vi "FolderMon start.vi"(4 "error in (no error)":errorcluster, 7 "daemon VI ref":refnum<vi>) -> (0 "error out":errorcluster, 3 "dup daemon VI ref":refnum<vi>)   [LabVIEW 2011]
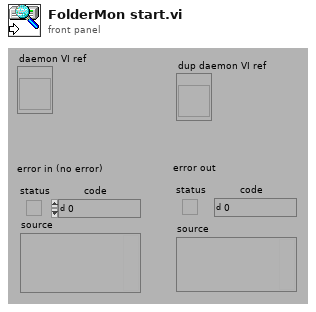
[diagram p1: front panel]
types:
  T1 = enum32{"Bad", "Idle", "Run top level", "Running"}
  T2 = typedef "Rendezvous RefNum" = refnum<k1>
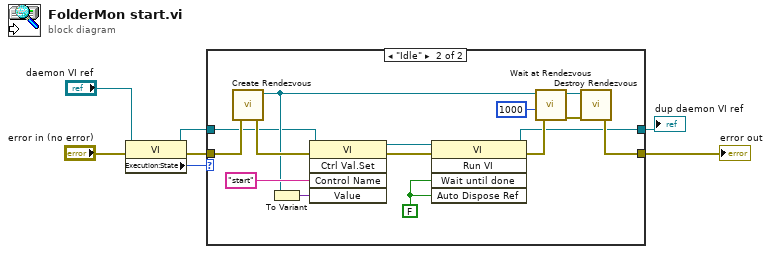
[diagram p0: block diagram]
diagram:
  n1 = property class="VI"(reference="daemon VI ref", error in="error in (no error)") -> (reference out=w5:refnum<vi>, error out=w7:errorcluster, "Execution:State"=w6:T1)
  n2 = case shown="\"Idle\"" w6 {
    tunnel: w7 -> [w8 w11]
    tunnel: [w8 w13] -> w1
    tunnel: w5 -> [w9 w10]
    tunnel: [w9 w12] -> w2
    frame "Bad", Default {
    }
    frame "Idle" {
      w20 = FALSE
      n3 = call <vilib>:"Create Rendezvous.vi"("error in (no error)"=w11) -> ("error out"=w19:errorcluster, "rendezvous"=w18:T2)  [unwired: 1 in, 4 out]
      n4 = To Variant(anything=w18) -> (Variant=w24:variant)
      n5 = invoke class="VI" method="Ctrl Val.Set"(reference=w10, error in=w19, "Control Name"="start", "Value"=w24) -> (reference out=w21:refnum<vi>, error out=w22:errorcluster)  [unwired: 1 in, 3 out]
      n6 = invoke class="VI" method="Run VI"(reference=w21, error in=w22, "Wait until done"=w20, "Auto Dispose Ref"=w20) -> (reference out=w12:refnum<vi>, error out=w17:errorcluster)  [unwired: 1 in, 3 out]
      n7 = call <vilib>:"Wait at Rendezvous.vi"("error in (no error)"=w17, "ms timeout (-1)"=1000, "rendezvous"=w18) -> ("error out"=w15:errorcluster, "rendezvous out"=w14:T2)  [unwired: 3 out]
      n8 = call <vilib>:"Destroy Rendezvous.vi"("error in (no error)"=w15, "rendezvous"=w14) -> ("error out"=w13:errorcluster)  [unwired: 5 out]
    }
  }
  "error out" <- w1
  "dup daemon VI ref" <- w2
